vi "GetLinksFromHTML.vi"(11 "SR XML in":string) -> (0 "Documents Used (B)":bool, 1 "Documents Used":string[][](array[string]), 2 "Documents Marked as Solution (B)":bool, 3 "Documents Marked as Solution":string[][](array[string]))   [LabVIEW 2017, in "DS_Lib.lvlib" / "SRNotesParser.lvlib"]
uses:
  SRNotesParser.lvlib
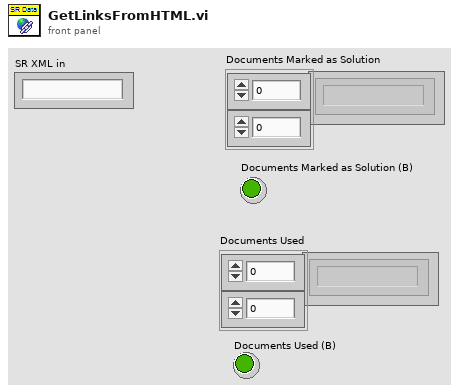
[diagram p1: front panel]
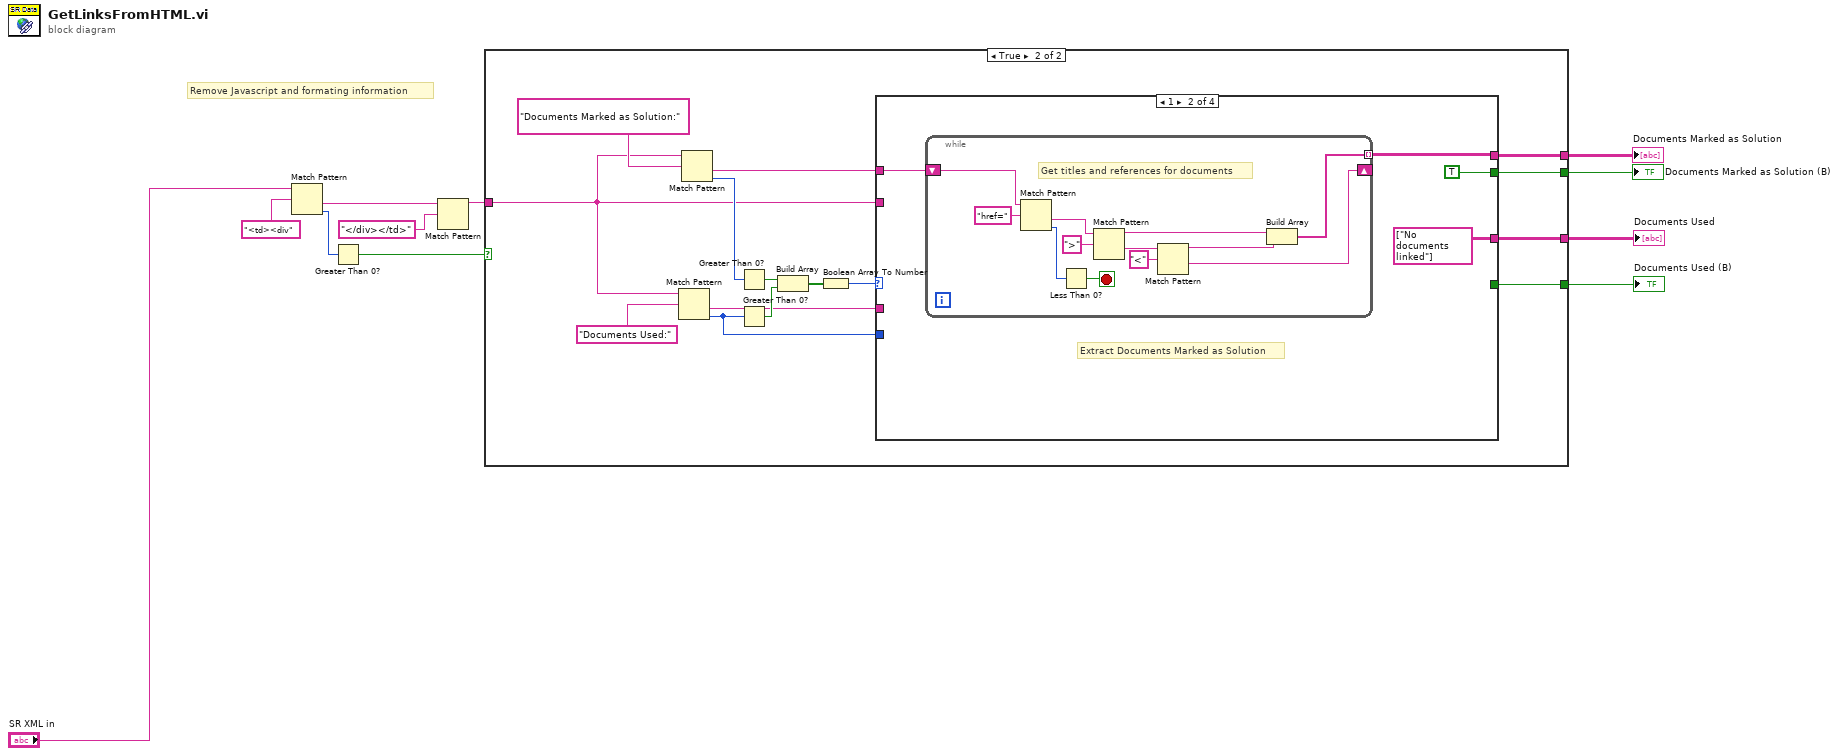
[diagram p0: block diagram]
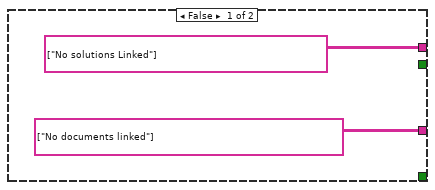
[diagram p2: hidden frame]
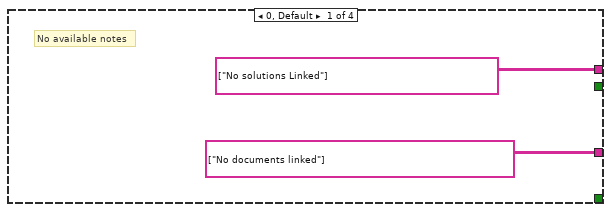
[diagram p3: hidden frame]
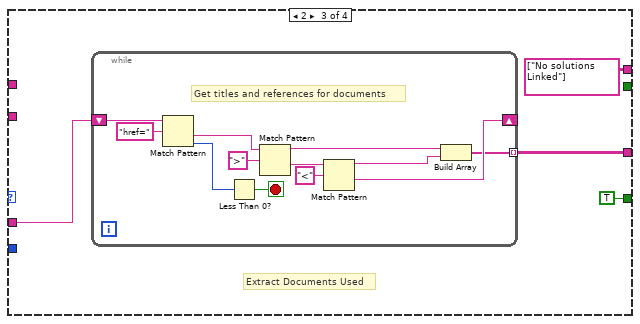
[diagram p4: hidden frame]
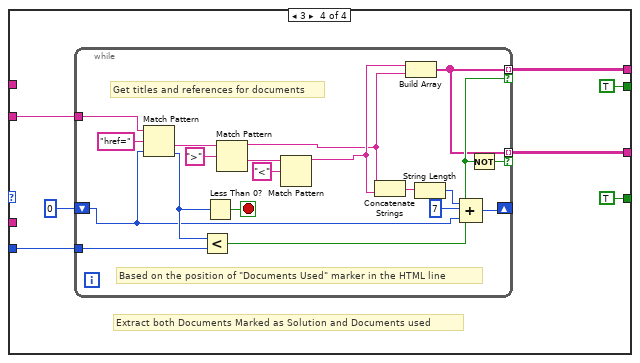
[diagram p5: hidden frame]
diagram:
  # "Remove Javascript and formating information"
  n1 = Match Pattern(string="SR XML in", regular expression="<td><div") -> (after substring=w9:string, offset past match=w7:i32)  [unwired: 1 in, 2 out]
  n2 = Greater Than 0?(x=w7) -> (x > 0?=w8:bool)
  n3 = Match Pattern(string=w9, regular expression="</div></td>") -> (before substring=w11:string)  [unwired: 1 in, 3 out]
  n4 = case shown="True" w8 {
    tunnel: w11 -> [_ w19]
    tunnel: [string[][] [["No solutions Linked"]] w17] -> w4
    tunnel: [string[][] [["No documents linked"]] w16] -> w3
    tunnel: [_ w15] -> w2
    tunnel: [_ w14] -> w1
    frame False {
    }
    frame True {
      n5 = Match Pattern(string=w19, regular expression="Documents Used:") -> (after substring=w20:string, offset past match=w18:i32)  [unwired: 1 in, 2 out]
      n6 = Match Pattern(string=w19, regular expression="Documents Marked as Solution:") -> (after substring=w22:string, offset past match=w27:i32)  [unwired: 1 in, 2 out]
      n7 = Greater Than 0?(x=w27) -> (x > 0?=w24:bool)
      n8 = Greater Than 0?(x=w18) -> (x > 0?=w25:bool)
      n9 = Build Array(w24, w25) -> (w23:bool[])
      n10 = Boolean Array To Number(Boolean array=w23) -> (number=w21:u32)
      n11 = case shown="1" w21 {
        tunnel: w22 -> [_ w34 _ _]
        tunnel: w20 -> [_ _ w50 _]
        tunnel: w19 -> [_ _ _ w69]
        tunnel: w18 -> [_ _ _ w68]
        tunnel: [string[][] [["No solutions Linked"]] w33 string[][] [["No solutions Linked"]] w66] -> w17
        tunnel: [string[][] [["No documents linked"]] string[][] [["No documents linked"]] w49 w65] -> w16
        tunnel: [_ TRUE _ TRUE] -> w15
        tunnel: [_ _ TRUE TRUE] -> w14
        frame 0, Default {
          # "No available notes"
        }
        frame 1 {
          # "Extract Documents Marked as Solution"
          n12 = while {
            shift-right: [w40] -> _
            shift-left: w34 -> [w45]
            tunnel: [w35] -> w33 mode=indexing
            stop <- w38 stop-if-true
            # "Get titles and references for documents"
            n13 = Match Pattern(string=w45, regular expression="href=") -> (after substring=w44:string, offset past match=w39:i32)  [unwired: 1 in, 2 out]
            n14 = Less Than 0?(x=w39) -> (x < 0?=w38:bool)
            n15 = Match Pattern(string=w44, regular expression=">") -> (before substring=w37:string, after substring=w42:string)  [unwired: 1 in, 2 out]
            n16 = Match Pattern(string=w42, regular expression="<") -> (before substring=w36:string, after substring=w40:string)  [unwired: 1 in, 2 out]
            n17 = Build Array(w37, w36) -> (w35:string[])
          }
        }
        frame 2 {
          # "Extract Documents Used"
          n18 = while {
            shift-right: [w56] -> _
            shift-left: w50 -> [w61]
            tunnel: [w51] -> w49 mode=indexing
            stop <- w55 stop-if-true
            # "Get titles and references for documents"
            n19 = Match Pattern(string=w61, regular expression="href=") -> (after substring=w60:string, offset past match=w54:i32)  [unwired: 1 in, 2 out]
            n20 = Less Than 0?(x=w54) -> (x < 0?=w55:bool)
            n21 = Match Pattern(string=w60, regular expression=">") -> (before substring=w53:string, after substring=w58:string)  [unwired: 1 in, 2 out]
            n22 = Match Pattern(string=w58, regular expression="<") -> (before substring=w52:string, after substring=w56:string)  [unwired: 1 in, 2 out]
            n23 = Build Array(w53, w52) -> (w51:string[])
          }
        }
        frame 3 {
          # "Extract both Documents Marked as Solution and Documents used"
          n24 = while {
            tunnel: [w70] -> w66 mode=indexing if=w81
            tunnel: w68 -> [w83]
            tunnel: [w70] -> w65 mode=indexing if=w82
            tunnel: w69 -> [w78]
            shift-right: [w74] -> _
            shift-left: 0 ("offset past match") -> [w73]
            stop <- w80 stop-if-true
            # "Based on the position of \"Documents Used\" marker in the HTML line"
            # "Get titles and references for documents"
            n25 = Match Pattern(string=w78, regular expression="href=", offset (0)=w73) -> (after substring=w87:string, offset past match=w79:i32)  [unwired: 2 out]
            n26 = Less?(x=w79, y=w83) -> (x < y?=w81:bool)
            n27 = Less Than 0?(x=w79) -> (x < 0?=w80:bool)
            n28 = Match Pattern(string=w87, regular expression=">") -> (before substring=w71:string, after substring=w85:string)  [unwired: 1 in, 2 out]
            n29 = Match Pattern(string=w85, regular expression="<") -> (before substring=w72:string)  [unwired: 1 in, 3 out]
            n30 = Concatenate Strings(w71, w72) -> (w77:string)
            n31 = Build Array(w72, w71) -> (w70:string[])
            n32 = String Length(string=w77) -> (length=w76:i32)
            n33 = Compound Arithmetic op=ADD(w76, 7 ("y"), w73) -> (w74:i32)
            n34 = Not(x=w81) -> (.not. x?=w82:bool)
          }
        }
      }
    }
  }
  "Documents Marked as Solution" <- w4
  "Documents Used" <- w3
  "Documents Marked as Solution (B)" <- w2
  "Documents Used (B)" <- w1
